vi "AcquireLock.vi"(8 "error in (no error)":errorcluster) -> (0 "error out":errorcluster)   [LabVIEW 2019]
uses:
  DataLock.vi
  Global.lvlib
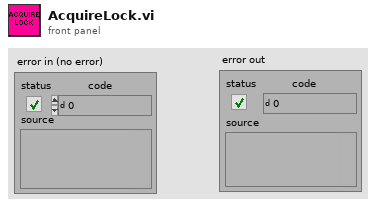
[diagram p1: front panel]
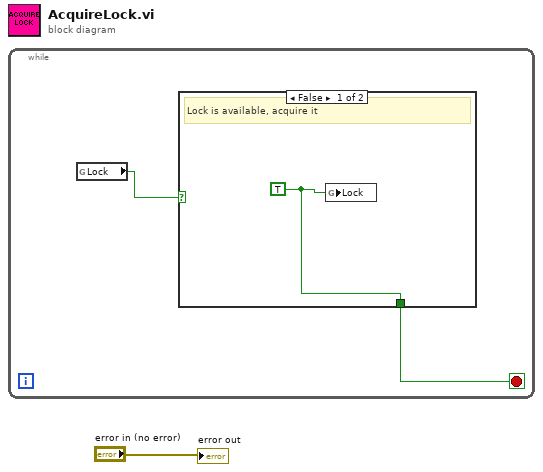
[diagram p0: block diagram]
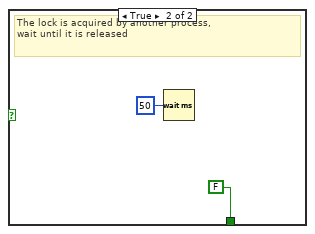
[diagram p2: hidden frame]
diagram:
  n1 = while {
    stop <- w2 stop-if-true
    n2 = global read "DataLock.vi" "Lock"() -> (w3:bool)
    n3 = case shown="False" w3 {
      tunnel: [w4 FALSE] -> w2
      frame False {
        w4 = TRUE ("Lock")
        # "Lock is available, acquire it"
        n4 = global write "DataLock.vi" "Lock"(w4) -> ()
      }
      frame True {
        # "The lock is acquired by another process, \nwait until it is released"
        n5 = Wait (ms)(milliseconds to wait=u32 50) -> ()  [unwired: 1 out]
      }
    }
  }
  "error out" <- "error in (no error)"
